vi "Hora.vi"() -> ()   [LabVIEW 2020]
panel:
  out "HORA UTC":i32
  out "HORA AM/PM":i32
  out "HORA MILITAR":i32
  out "SEGUNDOS":i32
  out "MINUTOS":i32
  in  "ENTRADA":string
  # "UTC"
  # "COLOMBIA"
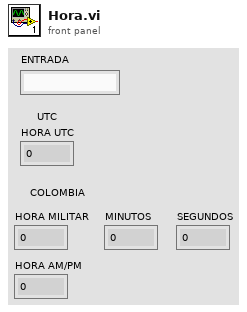
[diagram p1: front panel]
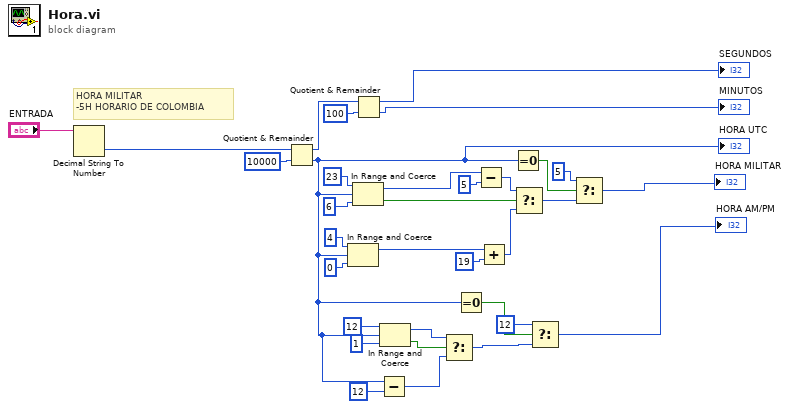
[diagram p0: block diagram]
diagram:
  # "HORA MILITAR \n-5H HORARIO DE COLOMBIA"
  n1 = Decimal String To Number(string="ENTRADA") -> (number=w24:i32)  [unwired: 2 in, 1 out]
  n2 = Quotient & Remainder(x=w24, y=10000) -> (x-y*floor(x/y)=w23:i32, floor(x/y)=w5:i32)
  "HORA UTC" <- w5
  n3 = In Range and Coerce(upper limit=4, x=w5, lower limit=0) -> (coerced(x)=w28:i32)  [unwired: 1 out]
  n4 = In Range and Coerce(upper limit=23, x=w5, lower limit=6) -> (coerced(x)=w26:i32, In Range?=w25:bool)
  n5 = Quotient & Remainder(x=w23, y=100) -> (x-y*floor(x/y)=→"SEGUNDOS":i32, floor(x/y)=→"MINUTOS":i32)
  n6 = Subtract(x=w5, y=12) -> (x-y=w6:i32)
  n7 = In Range and Coerce(upper limit=12, x=w5, lower limit=1) -> (coerced(x)=w8:i32, In Range?=w9:bool)
  n8 = Select(t=w8, s=w9, f=w6) -> (s? t:f=w3:i32)
  n9 = Equal To 0?(x=w5) -> (x = 0?=w4:bool)
  n10 = Subtract(x=w26, y=5) -> (x-y=w27:i32)
  n11 = Add(x=w28, y=19) -> (x+y=w29:i32)
  n12 = Equal To 0?(x=w5) -> (x = 0?=w31:bool)
  n13 = Select(t=w27, s=w25, f=w29) -> (s? t:f=w30:i32)
  n14 = Select(t=12, s=w4, f=w3) -> (s? t:f=→"HORA AM/PM":i32)
  n15 = Select(t=5, s=w31, f=w30) -> (s? t:f=→"HORA MILITAR":i32)
